vi "Register FKs.vi"(8 "error in (no error)":errorcluster, 11 "Panel Form Controller in":refnum<class "Panel Form Controller.lvclass">) -> (0 "error out":errorcluster, 3 "Panel Form Controller out":refnum<class "Panel Form Controller.lvclass">)   [LabVIEW 2020, in "Panel Form Controller.lvlib" / "Panel Form Controller.lvclass"]
uses:
  Panel Form Controller.lvclass
  C:/Program Files (x86)/National Instruments/LabVIEW 2020/vi.lib/ActorFramework/Actor/Actor.lvclass
  Forms Server/Update Fields Logic/Field FK PK Info.ctl
  <vilib>/ActorFramework/Actor/Actor.lvclass/Actor.ctl
  Panel Form Controller.lvclass/Panel Form Controller.ctl
  Forms Model/Form Model Interfaces/Form Model Messages Messages/Register FKs Msg/Register FKs Msg.lvclass/Register FKs Msg.ctl
  <vilib>/ActorFramework/Message Enqueuer/Message Enqueuer.lvclass/Message Enqueuer.ctl
  <vilib>/ActorFramework/Message Enqueuer/Enqueue.vi
  Database OOP/Table Libraries/Basic Form/Basic Form.lvclass
  C:/Users/User/Desktop/Raman Program/Database OOP/source/Database OOP/Table Libraries/Basic Table/Basic Table Class/Basic Table.lvclass
  Forms Model/Form Model Interfaces/Form Model Messages Messages/Register FKs Msg/Register FKs Msg.lvclass
  C:/Program Files (x86)/National Instruments/LabVIEW 2020/vi.lib/ActorFramework/Message/Message.lvclass
  <vilib>/ActorFramework/Message Priority Queue/Priority Enqueue.vi
  Database OOP/Table Libraries/Table Configuration Interface/Table Configuration Interface.lvclass
  Database OOP/Table Libraries/Basic Table/Basic Table Class/Basic Table.lvclass
  <vilib>/ActorFramework/Actor/Actor.lvclass
  Forms Server/Form Server Interfaces.lvlib
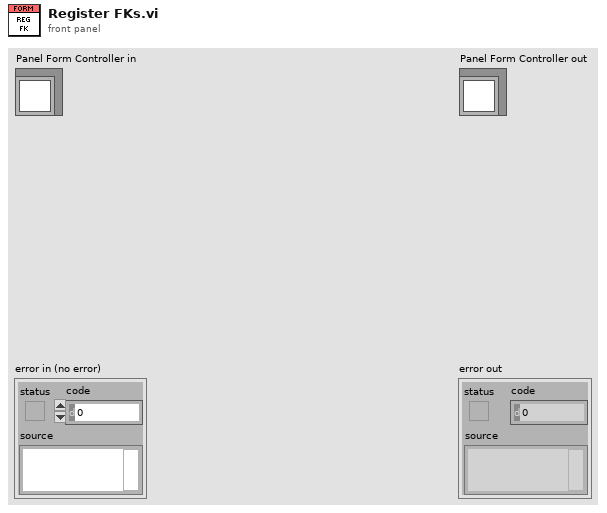
[diagram p1: front panel]
types:
  T1 = typedef "Form Server Interfaces.lvlib/Field FK PK Info.ctl" = cluster{"Field ID":string[], "FK Table":string[], "FK Column":string[], "PK Table":string[], "PK Column":string[]}
  T2 = typedef "Column Interfaces.lvlib/FK Info.ctl" = cluster{"PK Table":string, "PK Column":string, "PK Display Column":string}
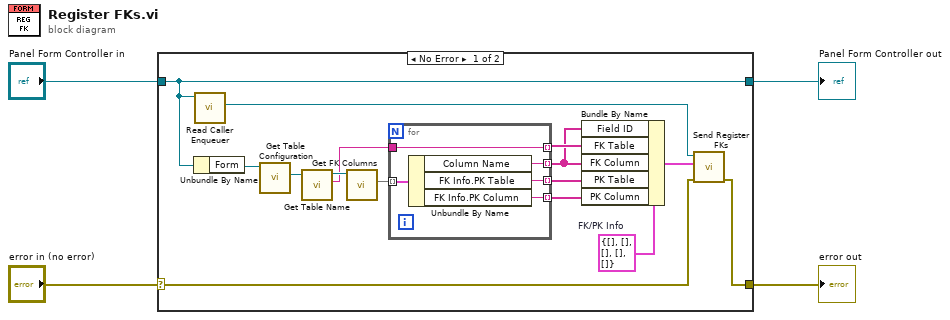
[diagram p0: block diagram]
diagram:
  n1 = case shown="No Error" "error in (no error)" {
    selector: "error in (no error)" -> [w6 w26]
    tunnel: [w5 w26] -> w3
    tunnel: [w18 w25] -> w1
    tunnel: "Panel Form Controller in" -> [w18 w25]
    frame No Error {
      w9 = T1 {"Field ID"=[], "FK Table"=[], "FK Column"=[], "PK Table"=[], "PK Column"=[]}  # FK/PK Info
      n2 = Unbundle By Name(w18) -> ("Form"=w19:refnum<class "Basic Form.lvclass">)
      n3 = call <vilib>:"Read Caller Enqueuer.vi"("Actor"=w18) -> ("Caller Enqueuer"=w7:refnum<class "Message Enqueuer.lvclass">)  [unwired: 10 in]
      n4 = call "Get Table Configuration.vi"("Basic Table in"=w19) -> ("Table Configuration"=w16:refnum<class "Table Configuration Interface.lvclass">)  [unwired: 8 in, 2 out]
      n5 = call-dynamic "Get Table Name.vi"("Table Configuration Interface in"=w16) -> ("Table Name"=w14:string, "Table Configuration Interface out"=w15:refnum<class "Table Configuration Interface.lvclass">)  [unwired: 8 in, 1 out]
      n6 = call-dynamic "Get FK Columns.vi"("Table Configuration Interface in"=w15) -> ("FKs"=w17:map{string, T2})  [unwired: 8 in, 2 out]
      n7 = for {
        tunnel: w17 -> [w24] mode=indexing
        tunnel: [w23] -> w10 mode=indexing
        tunnel: [w22] -> w12 mode=indexing
        tunnel: [w21] -> w11 mode=indexing
        tunnel: w14 -> [w20]
        tunnel: [w20] -> w13 mode=indexing
        n8 = Unbundle By Name(w24) -> ("Column Name"=w23:string, "FK Info.PK Table"=w22:string, "FK Info.PK Column"=w21:string)
      }
      n9 = Bundle By Name(cluster=w9, "Field ID"=w10, "FK Table"=w13, "FK Column"=w10, "PK Table"=w12, "PK Column"=w11) -> (w8:T1)
      n10 = call "Send Register FKs.vi"("error in (no error)"=w6, "FK/PK Info"=w8, "Message Enqueuer"=w7) -> ("error out"=w5:errorcluster)  [unwired: 7 in, 1 out]
    }
    frame Error {
    }
  }
  "error out" <- w3
  "Panel Form Controller out" <- w1
